vi "lab7.vi"() -> ()   [LabVIEW 2013]
uses:
  <vilib>/measure/NI_MABase.lvlib
  <vilib>/measure/NI_MAPro.lvlib
  <vilib>/measure/macond.llb/IIR Filter for 1 Chan.vi
  <vilib>/gmath/NI_Gmath.lvlib
  <vilib>/Analysis/NI_AALPro.lvlib
  <vilib>/Analysis/2dsp.llb/Power Spectrum (DBL).vi
  <vilib>/Analysis/4window.llb/Blackman Window (DBL).vi
  <vilib>/Analysis/4window.llb/Hamming Window (DBL).vi
  <vilib>/Analysis/4window.llb/Blackman-Harris Window (DBL).vi
  <vilib>/Analysis/4window.llb/Cosine Tapered Window (DBL).vi
  <vilib>/Analysis/3filter.llb/Filter Structure Type.ctl
  <vilib>/Analysis/NI_AALBase.lvlib
panel:
  in  "Amplitude":dbl=1.0 format="%.2p"
  in  "?":T1(tab)
  out "?":sgl[][](graph)
  out "Filtered Spectrum":dbl[](graph)
  out "Windowed Spectrum":dbl[](graph)
  out "Signal":waveform(dbl)(graph)
  out "Noise":waveform(dbl)(graph)
  out "Sig + noise":waveform(dbl)(graph)
  out "Filtered":waveform(dbl)(graph)
  in  "Window type":T2(ring)
  in  "filter structure option":T3=10 items=["IIR 2nd Order"=0, "IIR 4th Order"=1, "Auto Select"=10]
  in  "Filter specifications":T4={"Topology"=enum."Butterworth", "Type"=enum."Lowpass", "Order"=1, "Lower Fc"=100.0, "Upper Fc"=200.0, "PB Ripple"=1.0, "SB Attenuation"=60.0} {"PB Ripple" format="%0.2f"; "SB Attenuation" format="%0.2f"; "Lower Fc" format="%0.2p"; "Upper Fc" format="%0.2p"}
  in  "Amplitude":dbl
  in  "Delta freq":dbl
  in  "Start freq":dbl
  in  "Mean":dbl
  in  "Order":dbl
  in  "Reset Noise":bool
  in  "noise type":T5(ring)
  in  "Reset":bool
  in  "Offset":dbl
  in  "Square duty cycle, %":dbl
  in  "Amplitude":dbl
  in  "Phase":dbl
  in  "Frequncy":dbl
  in  "signal type":T6(ring)
  in  "?":bool
  # "Sine Wave parameters"
  # "Gamma noise parameters"
  # "Poisson noise parameters"
  # "Other Wave-types parameters"
  # "Multitone noise parameters"
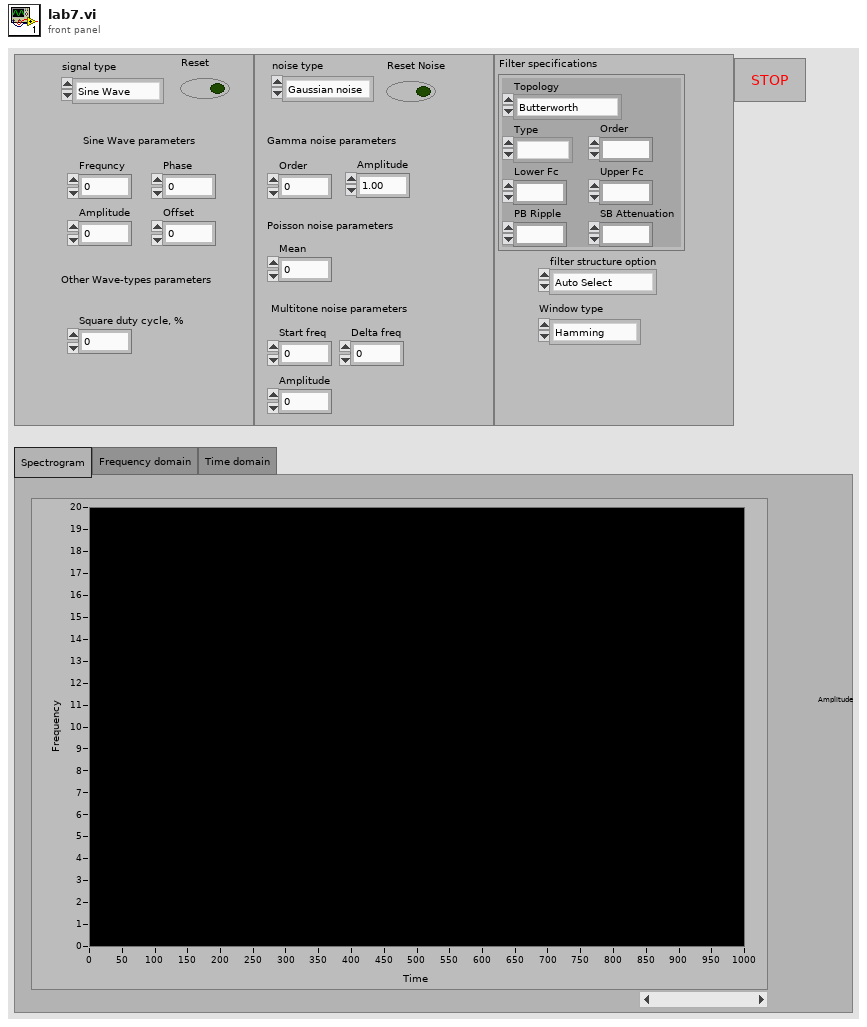
[diagram p1: front panel]
types:
  T1 = enum32{"Spectrogram", "Frequency domain", "Time domain"}
  T2 = enum16{"Hamming", "Blackman", "Blackman-Harris", "Tapered cos"}
  T3 = typedef "NI_AALBase.lvlib/Filter Structure Type.ctl" = u16
  T4 = cluster{"Topology":enum16{"Off", "Butterworth", "Chebyshev", "Inverse Chebyshev", "Elliptic", "Bessel"}, "Type":enum16{"Lowpass", "Highpass", "Bandpass", "Bandstop"}, "Order":i32, "Lower Fc":dbl, "Upper Fc":dbl, "PB Ripple":dbl, "SB Attenuation":dbl}
  T5 = enum16{"Gaussian noise", "Multitone Noise", "Gamma Noise", "Poisson Noise"}
  T6 = enum16{"Sine Wave", "Triangle Wave", "Square Wave", "Sawtooth Wave"}
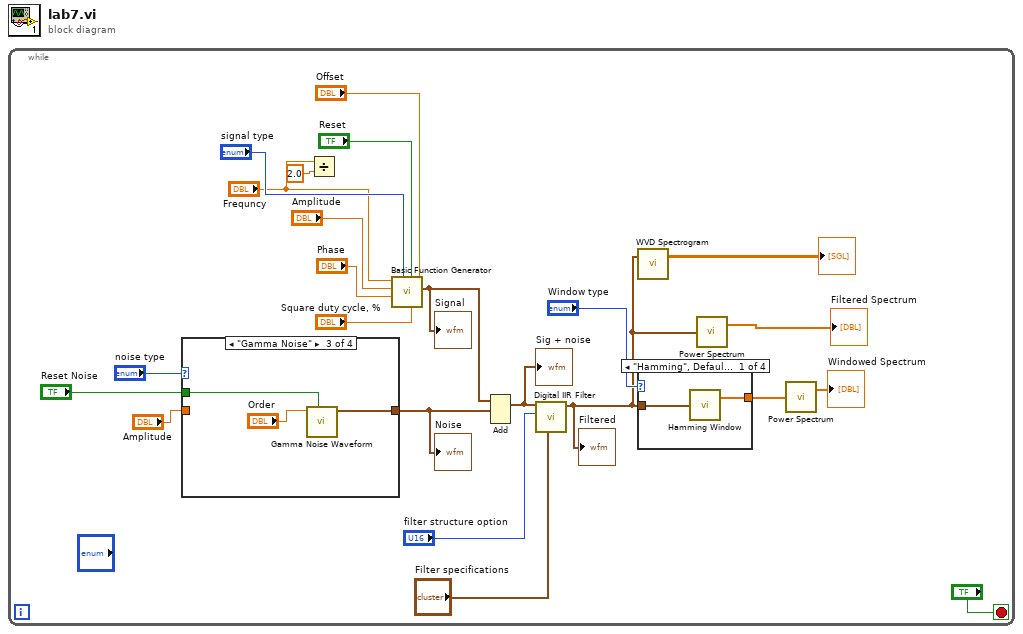
[diagram p0: block diagram]
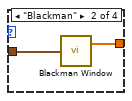
[diagram p2: hidden frame]
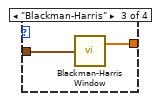
[diagram p3: hidden frame]
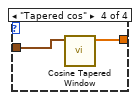
[diagram p4: hidden frame]
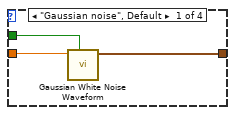
[diagram p5: hidden frame]
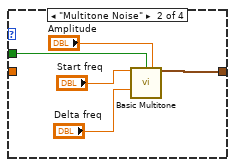
[diagram p6: hidden frame]
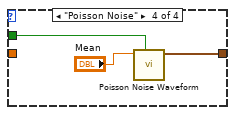
[diagram p7: hidden frame]
diagram:
  n1 = while {
    stop <- "?" stop-if-true
    n2 = case shown="\"Gamma Noise\"" "noise type" {
      tunnel: [w34 w38 w41 w43] -> w12
      tunnel: "Reset Noise" -> [w33 w39 w40 w45]
      tunnel: "Amplitude" -> [w32 _ _ _]
      frame "Gaussian noise", Default {
        n3 = call <vilib>:"Gaussian White Noise Waveform.vi"("reset signal"=w33, "standard deviation"=w32) -> ("signal out"=w34:waveform(dbl))  [unwired: 8 in, 1 out]
      }
      frame "Multitone Noise" {
        n4 = call <vilib>:"Basic Multitone.vi"("start frequency"="Start freq", "reset signal"=w39, "amplitude"="Amplitude", "delta frequency"="Delta freq") -> ("signal out"=w38:waveform(dbl))  [unwired: 8 in, 3 out]
      }
      frame "Gamma Noise" {
        n5 = call <vilib>:"Gamma Noise Waveform.vi"("reset signal"=w40, "order"="Order") -> ("signal out"=w41:waveform(dbl))  [unwired: 8 in, 1 out]
      }
      frame "Poisson Noise" {
        n6 = call <vilib>:"Poisson Noise Waveform.vi"("reset signal"=w45, "mean"="Mean") -> ("signal out"=w43:waveform(dbl))  [unwired: 8 in, 1 out]
      }
    }
    "Noise" <- w12
    n7 = Divide(x="Frequncy", y=2.0) -> ()  [unwired: 1 out]
    n8 = call <vilib>:"Basic Function Generator.vi"("offset"="Offset", "square wave duty cycle (%)"="Square duty cycle, %", "reset signal"="Reset", "signal type"="signal type", "phase"="Phase", "amplitude"="Amplitude", "frequency"="Frequncy") -> ("signal out"=w3:waveform(dbl))  [unwired: 2 in, 2 out]
    "Signal" <- w3
    n9 = Add(1:w12, 2:w3) -> (0:w2:waveform(dbl))  [unwired: 1 in, 1 out]
    "Sig + noise" <- w2
    n10 = call-poly <vilib>:"Digital IIR Filter.vi"("IIR filter specifications"="Filter specifications", "filter structure option"="filter structure option", "signal in"=w2) -> ("signal out"=w6:waveform(dbl))  [unwired: 6 in, 2 out]
    "Filtered" <- w6
    n11 = call <vilib>:"WVD Spectrogram.vi"("X"=w6) -> ("WVD Spectrogram {X}"=→"?":sgl[][])  [unwired: 1 in, 1 out]
    n12 = case shown="\"Hamming\", Default" "Window type" {
      tunnel: w6 -> [w25 w27 w29 w31]
      tunnel: [w24 w26 w28 w30] -> w5
      frame "Hamming", Default {
        n13 = call-poly <vilib>:"Hamming Window.vi"("X"=w25) -> ("Windowed X"=w24:dbl[])  [unwired: 1 out]
      }
      frame "Blackman" {
        n14 = call-poly <vilib>:"Blackman Window.vi"("X"=w27) -> ("Windowed X"=w26:dbl[])  [unwired: 1 out]
      }
      frame "Blackman-Harris" {
        n15 = call-poly <vilib>:"Blackman-Harris Window.vi"("X"=w29) -> ("Windowed X"=w28:dbl[])  [unwired: 1 out]
      }
      frame "Tapered cos" {
        n16 = call-poly <vilib>:"Cosine Tapered Window.vi"("X"=w31) -> ("Windowed X"=w30:dbl[])  [unwired: 9 in, 1 out]
      }
    }
    n17 = call-poly <vilib>:"Power Spectrum.vi"("X"=w6) -> ("Power Spectrum"=→"Filtered Spectrum":dbl[])  [unwired: 1 out]
    n18 = call-poly <vilib>:"Power Spectrum.vi"("X"=w5) -> ("Power Spectrum"=→"Windowed Spectrum":dbl[])  [unwired: 1 out]
  }
